vi "v3.vi"   [LabVIEW 2023]
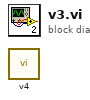
[diagram p0: block diagram]
diagram:
  n1 = call "v4.vi"() -> ()  [unwired: 12 in]
